vi "saveData.vi"(4 "type":enum16{"ascii", "binary"}(ring), 5 "file name":string, 6 "이미지 저장 VI":refnum<vi>, 7 "file path 경로":path, 8 "error in":errorcluster caption="에러 입력", 9 "body":string[][](array[string]), 10 "header":string[][](array[string]), 11 "Function":T1) -> (0 "error out":errorcluster caption="에러 출력", 1 "경로":path, 3 "ref":i32)   [LabVIEW 2018]
uses:
  control/enumFgvFunction.ctl
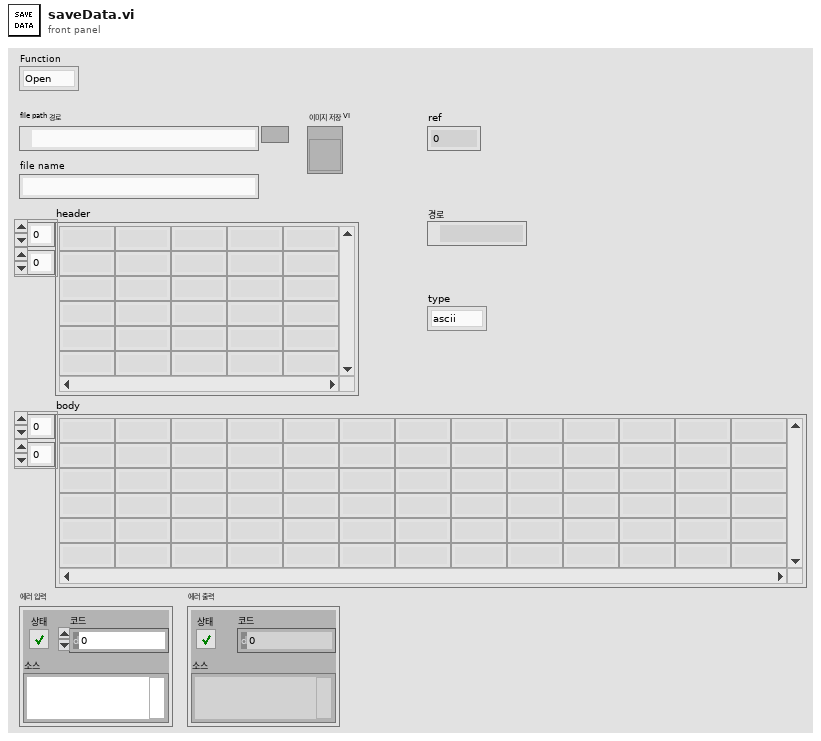
[diagram p1: front panel]
types:
  T1 = typedef "enumFgvFunction.ctl" = enum16{"Open", "Read", "Check", "Write", "Close"}
  T2 = enum16{"open", "replace", "create", "open or create", "replace or create", "replace or create with confirmation"}
  T3 = typedef "imagedata.ctl" = cluster{"image type":i32, "image depth":i32, "image":u8[], "mask":u8[], "colors":u32[], "Rectangle":cluster{"left":i16, "top":i16, "right":i16, "bottom":i16}}
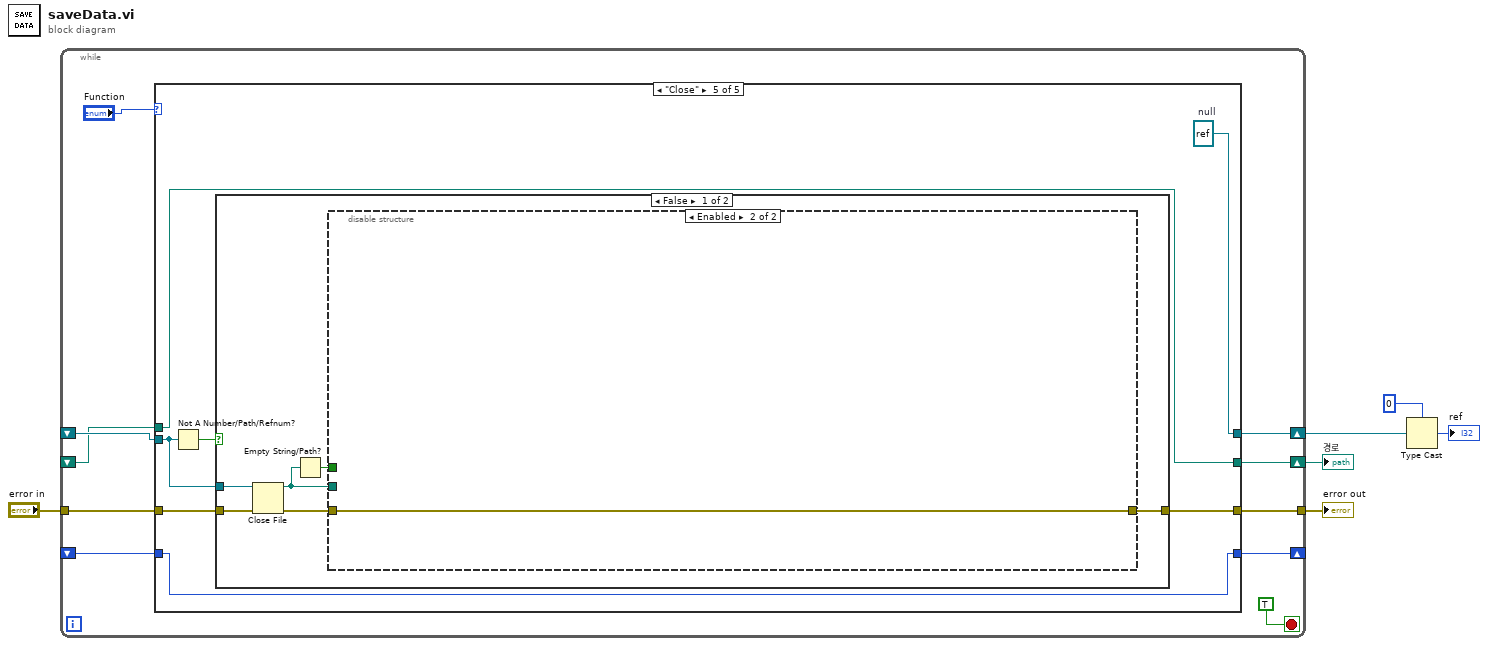
[diagram p0: block diagram]
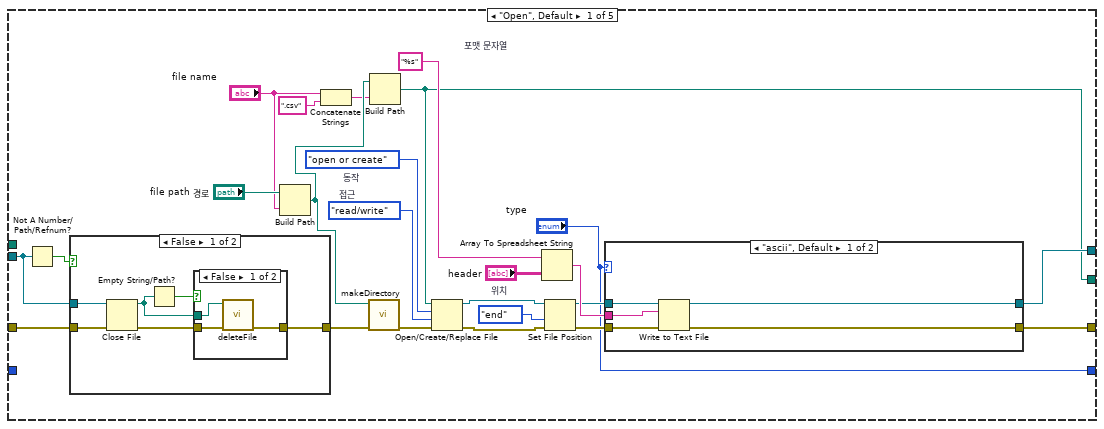
[diagram p2: hidden frame]
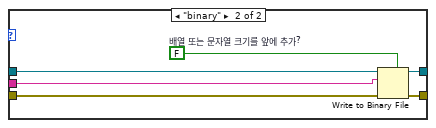
[diagram p3: hidden frame]
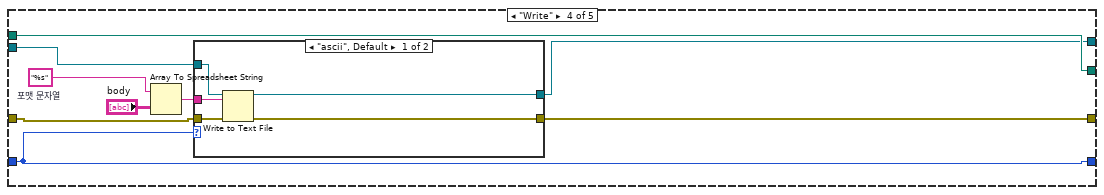
[diagram p8: hidden frame]
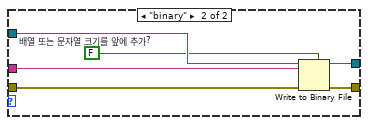
[diagram p9: hidden frame]
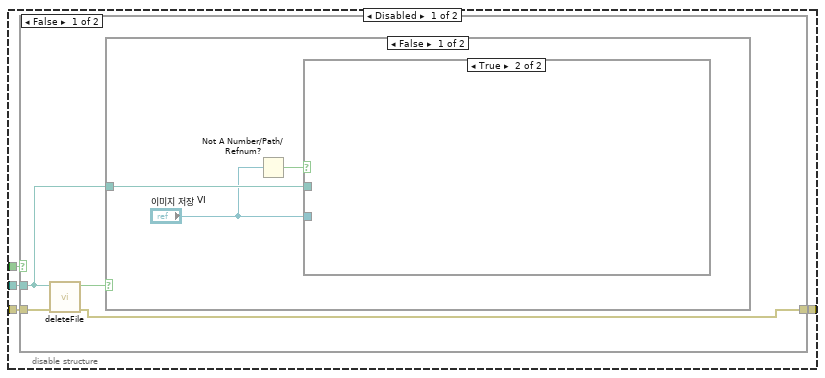
[diagram p10: hidden frame]
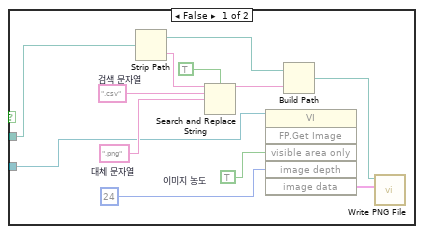
[diagram p11: hidden frame]
diagram:
  n1 = while {
    shift-right: [w12] -> w2
    shift-left: _ -> [w15]
    tunnel: "error in" -> [w14]
    tunnel: [w13] -> w5
    shift-right: [w11] -> w1
    shift-left: _ -> [w10]
    shift-right: [w9] -> _
    shift-left: _ -> [w8]
    stop <- TRUE stop-if-true
    n2 = case shown="\"Close\"" "Function" {
      tunnel: [w40 w66 w69 w73 w97] -> w12
      tunnel: w15 -> [w36 w66 w69 w79 w93]
      tunnel: w14 -> [w38 w65 w70 w78 w96]
      tunnel: [w39 w65 w70 w74 w95] -> w13
      tunnel: [w20 w64 w68 w75 w92] -> w11
      tunnel: w10 -> [_ w64 w68 w75 w92]
      tunnel: w8 -> [_ w63 w67 w71 w91]
      tunnel: ["type" w63 w67 w71 w91] -> w9
      frame "Open", Default {
        w29 = "%s"  # 포맷 문자열
        w28 = enum16{"read/write", "read-only", "write-only"}."read/write"  # 접근
        w27 = T2."open or create"  # 동작
        w26 = enum16{"start", "end", "current"}."end"  # 위치
        n3 = Not A Number/Path/Refnum?(number/path/refnum=w36) -> (NaN/Path/Refnum?=w37:bool)
        n4 = case shown="False" w37 {
          tunnel: w38 -> [w57 w62]
          tunnel: [w52 w62] -> w19
          tunnel: w36 -> [w56 _]
          frame False {
            n5 = Close File(refnum=w56, error in=w57) -> (path=w54:path, error out=w53:errorcluster)
            n6 = Empty String/Path?(string/path=w54) -> (empty?=w55:bool)
            n7 = case shown="False" w55 {
              tunnel: w54 -> [w60 _]
              tunnel: w53 -> [w59 w61]
              tunnel: [w58 w61] -> w52
              frame False {
                n8 = call "deleteFile.vi"("에러 입력"=w59, "파일 경로"=w60) -> ("에러 출력"=w58:errorcluster)  [unwired: 8 in, 1 out]
              }
              frame True {
              }
            }
          }
          frame True {
          }
        }
        n9 = Build Path(base path="file path 경로", name or relative path="file name") -> (appended path=w24:path)
        n10 = Concatenate Strings("file name", ".csv") -> (w21:string)
        n11 = call "makeDirectory.vi"("error in"=w19, "파일저장경로"=w24) -> ("error out"=w18:errorcluster)  [unwired: 9 in]
        n12 = Build Path(base path=w24, name or relative path=w21) -> (appended path=w20:path)
        n13 = Open/Create/Replace File(file path (use dialog)=w20, error in=w18, operation (0:open)=w27, access (0:read/write)=w28) -> (refnum out=w34:refnum<file>, error out=w33:errorcluster)  [unwired: 2 in, 1 out]
        n14 = Array To Spreadsheet String(array="header", 3:w29) -> (spreadsheet string=w35:string)  [unwired: 1 in]
        n15 = Set File Position(refnum=w34, from (0:start)=w26, error in=w33) -> (refnum out=w31:refnum<file>, error out=w32:errorcluster)  [unwired: 1 in]
        n16 = case shown="\"ascii\", Default" "type" {
          tunnel: [w45 w48] -> w40
          tunnel: [w44 w50] -> w39
          tunnel: w35 -> [w43 w47]
          tunnel: w32 -> [w42 w51]
          tunnel: w31 -> [w41 w49]
          frame "ascii", Default {
            n17 = Write to Text File(file (use dialog)=w41, text=w43, error in=w42) -> (refnum out=w45:refnum<file>, error out=w44:errorcluster)  [unwired: 1 in, 1 out]
          }
          frame "binary" {
            w46 = FALSE  # 배열 또는 문자열 크기를 앞에 추가?
            n18 = Write to Binary File(file (use dialog)=w49, data=w47, error in=w51, 5:w46) -> (refnum out=w48:refnum<file>, error out=w50:errorcluster)  [unwired: 2 in, 1 out]
          }
        }
      }
      frame "Read" {
      }
      frame "Check" {
      }
      frame "Write" {
        w77 = "%s"  # 포맷 문자열
        n19 = Array To Spreadsheet String(array="body", 3:w77) -> (spreadsheet string=w72:string)  [unwired: 1 in]
        n20 = case shown="\"ascii\", Default" w71 {
          tunnel: [w84 w87] -> w73
          tunnel: [w83 w89] -> w74
          tunnel: w72 -> [w82 w86]
          tunnel: w78 -> [w81 w90]
          tunnel: w79 -> [w80 w88]
          frame "ascii", Default {
            n21 = Write to Text File(file (use dialog)=w80, text=w82, error in=w81) -> (refnum out=w84:refnum<file>, error out=w83:errorcluster)  [unwired: 1 in, 1 out]
          }
          frame "binary" {
            w85 = FALSE  # 배열 또는 문자열 크기를 앞에 추가?
            n22 = Write to Binary File(file (use dialog)=w88, data=w86, error in=w90, 5:w85) -> (refnum out=w87:refnum<file>, error out=w89:errorcluster)  [unwired: 2 in, 1 out]
          }
        }
      }
      frame "Close" {
        w97 = refnum<file> refnum  # null
        n23 = Not A Number/Path/Refnum?(number/path/refnum=w93) -> (NaN/Path/Refnum?=w94:bool)
        n24 = case shown="False" w94 {
          tunnel: w96 -> [w100 w129]
          tunnel: [w99 w129] -> w95
          tunnel: w93 -> [w98 _]
          frame False {
            n25 = Close File(refnum=w98, error in=w100) -> (path=w101:path, error out=w102:errorcluster)
            n26 = Empty String/Path?(string/path=w101) -> (empty?=w103:bool)
            n27 = disable-structure shown="Enabled" {
              disable-tunnel: w103 -> [w107 _]
              disable-tunnel: w102 -> [w106 w128]
              disable-tunnel: w101 -> [w105 _]
              disable-tunnel: [w104 w128] -> w99
              frame Disabled {
                n28 = case shown="False" w107 {
                  tunnel: w105 -> [w109 _]
                  tunnel: w106 -> [w110 w127]
                  tunnel: [w111 w127] -> w104
                  frame False {
                    n29 = call "deleteFile.vi"("에러 입력"=w110, "파일 경로"=w109) -> ("에러 출력"=w111:errorcluster, "deleted"=w108:bool)  [unwired: 8 in]
                    n30 = case shown="False" w108 {
                      tunnel: w109 -> [w114 _]
                      frame False {
                        n31 = Not A Number/Path/Refnum?(number/path/refnum="이미지 저장 VI") -> (NaN/Path/Refnum?=w112:bool)
                        n32 = case shown="True" w112 {
                          tunnel: w114 -> [w117 _]
                          tunnel: "이미지 저장 VI" -> [w116 _]
                          frame False {
                            w115 = 24  # 이미지 농도
                            w118 = ".png"  # 대체 문자열
                            w119 = ".csv"  # 검색 문자열
                            n33 = Strip Path(path=w117) -> (stripped path=w124:path, name=w123:string)
                            n34 = Search and Replace String(case sensitive?=TRUE ("대소문자 구분 무시?"), input string=w123, search string=w119, replace string=w118) -> (result string=w122:string)  [unwired: 4 in, 3 out]
                            n35 = invoke on="인보크 노드" class="VI" method="FP.Get Image"(reference=w116, "visible area only"=TRUE ("보이기 영역만"), "image depth"=w115) -> ("image data"=w125:T3)  [unwired: 3 in, 5 out]
                            n36 = Build Path(base path=w124, name or relative path=w122) -> (appended path=w126:path)
                            n37 = call <vilib>:"Write PNG File.vi"("image data"=w125, "path to PNG file"=w126) -> ()  [unwired: 8 in, 2 out]
                          }
                          frame True {
                          }
                        }
                      }
                      frame True {
                      }
                    }
                  }
                  frame True {
                  }
                }
              }
              frame Enabled {
              }
            }
          }
          frame True {
          }
        }
      }
    }
  }
  "error out" <- w5
  "경로" <- w1
  n38 = Type Cast(type=0, x=w2) -> (*(type *) &x=→"ref":i32)
